vi "Test MQTT-3.1.2-1.vi"(8 "error in (no error)":errorcluster) -> (0 "error out":errorcluster)   [LabVIEW 2013]
uses:
  source/Server/Connection/TCPConnection.lvclass
  <vilib>/LabVIEW Open Source Project/MQTT Control Packets/Control Packets/CONNECT/CONNECT.lvclass
  <vilib>/LabVIEW Open Source Project/MQTT Control Packets/Control Packets/ControlPacket/ControlPacket.lvclass
  <vilib>/addons/_JKI Toolkits/Caraya/classes/Test/Test.lvclass
  <vilib>/addons/_JKI Toolkits/Caraya/classes/Assert/Assert.lvclass
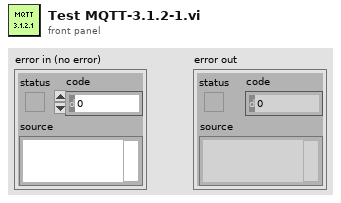
[diagram p1: front panel]
types:
  T1 = enum16{"Standard", "Buffered", "CRLF", "Immediate"}
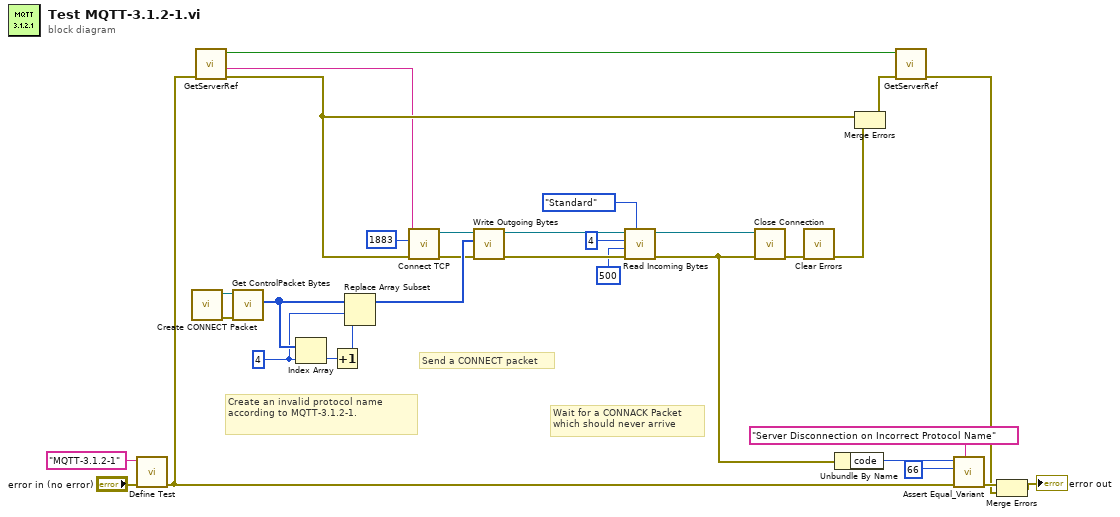
[diagram p0: block diagram]
diagram:
  w26 = 4 ("index")
  # "Wait for a CONNACK Packet\nwhich should never arrive"
  # "Create an invalid protocol name according to MQTT-3.1.2-1."
  # "Send a CONNECT packet"
  n1 = call <vilib>:"Define Test.vi"("error in (no error)"="error in (no error)", "Label (VI Title)"="MQTT-3.1.2-1") -> ("error out"=w5:errorcluster)  [unwired: 9 in]
  n2 = call <vilib>:"Create CONNECT Packet.vi"() -> ("error out"=w31:errorcluster, "CONNECT"=w32:refnum<class "CONNECT.lvclass">)  [unwired: 10 in]
  n3 = call "GetServerRef.vi"("error in"=w5) -> ("error out"=w4:errorcluster, "Server address"=w1:string, "Created"=w6:bool)  [unwired: 7 in, 1 out]
  n4 = call <vilib>:"Get ControlPacket Bytes.vi"("error in (no error)"=w31, "ControlPacket"=w32) -> ("Bytes Stream"=w28:u8[])  [unwired: 6 in, 3 out]
  n5 = Index Array(array=w28, index=w26) -> (element=w11:u8)
  n6 = Increment(x=w11) -> (x+1=w10:u8)
  n7 = Replace Array Subset(array=w28, new element=w10, index=w26) -> (w27:u8[])
  n8 = call "Connect TCP.vi"("error in (no error)"=w4, "remote port (80)"=u16 1883, "address (localhost)"=w1) -> ("error out"=w7:errorcluster, "TCPConnection out"=w8:refnum<class "TCPConnection.lvclass">)  [unwired: 7 in]
  n9 = call "Write Outgoing Bytes.vi"("error in (no error)"=w7, "Bytes"=w27, "TCPConnection in"=w8) -> ("error out"=w29:errorcluster, "TCPConnection out"=w30:refnum<class "TCPConnection.lvclass">)  [unwired: 7 in]
  n10 = call "Read Incoming Bytes.vi"("mode (standard)"=T1."Standard", "error in (no error)"=w29, "timeout (1000 ms)"=500 ("timeout ms (25000)"), "bytes to read (100)"=4 ("bytes to read"), "TCPConnection in"=w30) -> ("error out"=w13:errorcluster, "TCPConnection out"=w25:refnum<class "TCPConnection.lvclass">)  [unwired: 3 in, 2 out]
  n11 = call-dynamic "Close Connection.vi"("error in (no error)"=w13, "TCPConnection in"=w25) -> ("error out"=w18:errorcluster)  [unwired: 8 in, 1 out]
  n12 = call <vilib>:"Clear Errors.vi"("error in (no error)"=w18) -> ("error out"=w12:errorcluster)  [unwired: 6 in]
  n13 = Unbundle By Name(w13) -> ("code"=w20:i32)
  n14 = Merge Errors(w4, w12) -> (w3:errorcluster)
  n15 = call "GetServerRef.vi"("error in"=w3, "Destroy (F)"=w6) -> ("error out"=w2:errorcluster)  [unwired: 6 in, 3 out]
  n16 = call <vilib>:"Assert Equal_Variant.vi"("Label"="Server Disconnection on Incorrect Protocol Name", "error in (no error)"=w5, "Y"=66 ("code"), "X"=w20) -> ("error out"=w23:errorcluster)  [unwired: 7 in]
  n17 = Merge Errors(w23, w2) -> (→"error out":errorcluster)
